vi "FlatToRichniswitch_grpc_ScanRequest.vi"(5 "OutputClusterType":T1, 11 "InputCluster":T3) -> (3 "OutputCluster":T1)   [LabVIEW 2021, in "NI Switch_client.lvlib"]
uses:
  NI Switch_client.lvlib
  niswitch_grpc_ScanRequest_initiation_enum/niswitch_grpc_ScanRequest_initiation_enum.lvclass
  nidevice_grpc_Session.ctl
  niswitch_grpc_ScanRequest.ctl
  niswitch_grpc_HandshakingInitiation.ctl
  nidevice_grpc_Session_Flat.ctl
  niswitch_grpc_ScanRequest_Flat.ctl
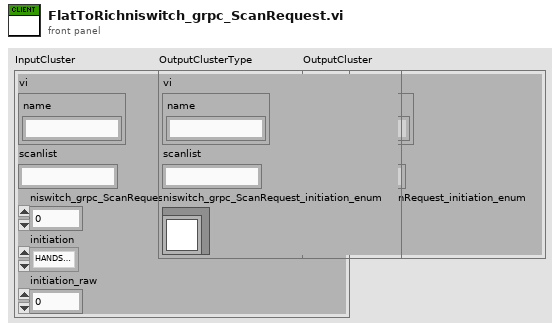
[diagram p1: front panel]
types:
  T1 = typedef "NI Switch_client.lvlib/niswitch_grpc_ScanRequest.ctl" = cluster{"vi":T2, "scanlist":string, "niswitch_grpc_ScanRequest_initiation_enum":refnum<class "niswitch_grpc_ScanRequest_initiation_enum.lvclass">}
  T2 = typedef "NI Switch_client.lvlib/nidevice_grpc_Session.ctl" = cluster{"name":string}
  T3 = typedef "NI Switch_client.lvlib/niswitch_grpc_ScanRequest_Flat.ctl" = cluster{"vi":T4, "scanlist":string, "niswitch_grpc_ScanRequest_initiation_enum_selected_index":i32, "initiation":T5, "initiation_raw":i32}
  T4 = typedef "NI Switch_client.lvlib/nidevice_grpc_Session_Flat.ctl" = cluster{"name":string}
  T5 = typedef "NI Switch_client.lvlib/niswitch_grpc_HandshakingInitiation.ctl" = enum32{"HANDSHAKING_INITIATION_NISWITCH_VAL_MEASUREMENT_DEVICE_INITIATED", "HANDSHAKING_INITIATION_NISWITCH_VAL_SWITCH_INITIATED"}
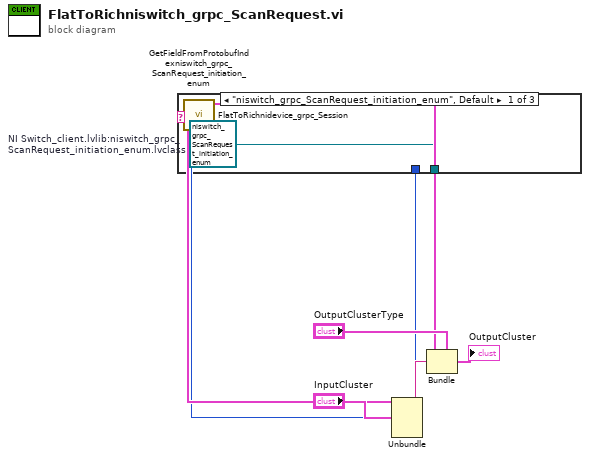
[diagram p0: block diagram]
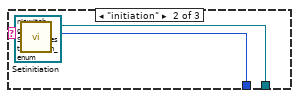
[diagram p2: hidden frame]
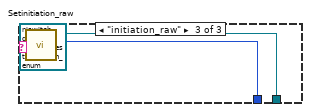
[diagram p3: hidden frame]
diagram:
  n1 = Unbundle "Unbundle"("InputCluster") -> ("vi"=w8:T4, "scanlist"=w6:string, "niswitch_grpc_ScanRequest_initiation_enum_selected_index"=w5:i32, "initiation"=w2:T5, "initiation_raw"=w1:i32)
  n2 = call "GetFieldFromProtobufIndexniswitch_grpc_ScanRequest_initiation_enum.vi"("protobuf index"=w5) -> ("oneof field name"=w4:string)
  n3 = case "niswitch_grpc_ScanRequest_initiation_enum" shown="\"niswitch_grpc_ScanRequest_initiation_enum\", Default" w4 {
    tunnel: [w12 w14 w17] -> w3
    tunnel: w2 -> [_ w15 _]
    tunnel: w1 -> [_ _ w18]
    frame "niswitch_grpc_ScanRequest_initiation_enum", Default {
      w12 = refnum<class "niswitch_grpc_ScanRequest_initiation_enum.lvclass"> refnum  # NI Switch_client.lvlib:niswitch_grpc_ScanRequest_initiation_enum.lvclass
    }
    frame "initiation" {
      n4 = call "Setinitiation.vi"("Set_Val"=w15, "OneOfTemplate in"=refnum<class "niswitch_grpc_ScanRequest_initiation_enum.lvclass"> refnum) -> ("OneOfTemplate out"=w14:refnum<class "niswitch_grpc_ScanRequest_initiation_enum.lvclass">)  [unwired: 8 in, 1 out]
    }
    frame "initiation_raw" {
      n5 = call "Setinitiation_raw.vi"("Set_Val"=w18, "OneOfTemplate in"=refnum<class "niswitch_grpc_ScanRequest_initiation_enum.lvclass"> refnum) -> ("OneOfTemplate out"=w17:refnum<class "niswitch_grpc_ScanRequest_initiation_enum.lvclass">)  [unwired: 8 in, 1 out]
    }
  }
  n6 = call "FlatToRichnidevice_grpc_Session.vi"("InputCluster"=w8) -> ("OutputCluster"=w7:T2)  [unwired: 10 in]
  n7 = Bundle "Bundle"(cluster="OutputClusterType", "vi"=w7, "scanlist"=w6, "niswitch_grpc_ScanRequest_initiation_enum"=w3) -> (→"OutputCluster":T1)
